vi "subVI_CurrentSourcing.vi"(4 "error in":errorcluster caption="에러 입력", 5 "stop (T)":bool=TRUE caption="정지(T)", 6 "timeout (s)":dbl=10.0 caption="타임아웃(초)" format="%0.2f", 7 "Curr set val":dbl[](array[numeric]) caption="배열" format="%0.2f") -> (0 "error out":errorcluster caption="에러 출력", 3 "task out":refnum<k21> caption="태스크 출력")   [LabVIEW 2016]
doc: "NI-DAQmx를 사용하여 태스크를 생성, 편집, 실행합니다. NI-DAQmx가 지원하는 디바이스의 완전한 리스트는 NI-DAQ Readme를 참조하십시오.\n\n이 익스프레스 VI를 블록다이어그램에 놓으면 DAQ 어시스턴트가 시작되어 새로운 태스크를 생성합니다, 태스크를 생성한 후, DAQ 어시스턴트 익스프레스 VI를 더블 클릭하여 해당 태스크를 편집할 수 있습니다. 연속적인 측정 또는 생성을 위해서는 DAQ 어시스턴트 익스프레스 주위에 while 루프를 놓습니다.\n\n연속적인 단일 포인트 입력 또는 출력의 경우 DAQ 어시스턴트 익스프레스 VI는 최적의 성능을 제공하지 않을 수도 있습니다. 높은 성능을 가진 단일 포인트 I/O 어플리케이션을 생성하는 기술에 대한 예제는 examples\\DAQmx\\Analog In\\Measure Voltage.llb의 Cont Acq&Graph Voltage-Single Point Optimization VI를 참조하십시오."
uses:
  <vilib>/DAQmx/write.llb/DAQmx Write.vi
  <vilib>/DAQmx/write.llb/DAQmx Write (Analog 1D DBL NChan 1Samp).vi
  <vilib>/DAQmx/create/channels.llb/DAQmx Create Channel (AO-Current-Basic).vi
  <vilib>/DAQmx/miscellaneous.llb/DAQmx Fill In Error Info.vi
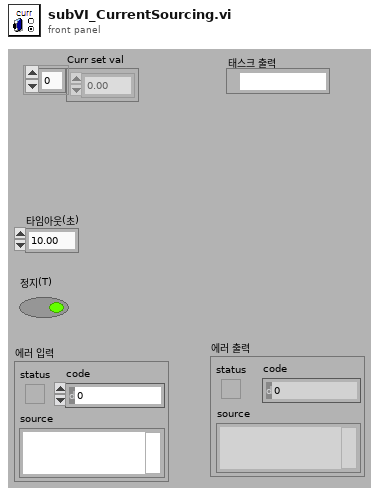
[diagram p1: front panel]
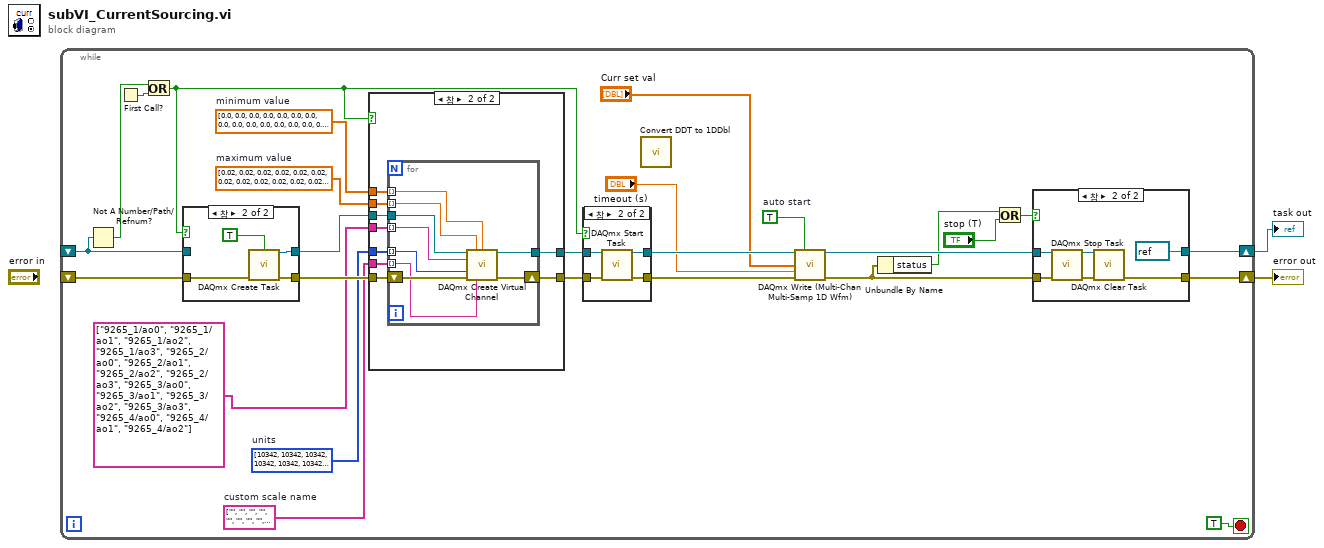
[diagram p0: block diagram]
diagram:
  n1 = while {
    shift-right: [w11] -> w1
    shift-left: _ -> [w26]
    shift-right: [w9] -> w2
    shift-left: _ -> [w27]
    stop <- TRUE stop-if-true
    w13 = TRUE  # auto start
    w19 = string[] ["", "", "", "", "", "", "", "", "", "", "", "", "", "", "", ""]  # custom scale name
    w20 = i32[] [10342, 10342, 10342, 10342, 10342, 10342, 10342, 10342, 10342, 10342, 10342, 10342, 10342, 10342, 10342, 10342] items=["Amps"=10342, "From Custom Scale"=10065]  # units
    w21 = dbl[] [0.02, 0.02, 0.02, 0.02, 0.02, 0.02, 0.02, 0.02, 0.02, 0.02, 0.02, 0.02, 0.02, 0.02, 0.02, 0.02]  # maximum value
    w22 = dbl[] [0.0, 0.0, 0.0, 0.0, 0.0, 0.0, 0.0, 0.0, 0.0, 0.0, 0.0, 0.0, 0.0, 0.0, 0.0, 0.0]  # minimum value
    n2 = Not A Number/Path/Refnum?(number/path/refnum=w26) -> (NaN/Path/Refnum?=w25:bool)
    n3 = First Call?() -> (First Call?: T/F=w28:bool)
    n4 = Or(x=w25, y=w28) -> (x .or. y?=w18:bool)
    n5 = case "케이스 구조" shown="참" w18 {
      tunnel: [w65 w69] -> w24
      tunnel: w26 -> [w65 _]
      tunnel: [w64 w68] -> w23
      tunnel: w27 -> [w64 w66]
      frame False {
      }
      frame True {
        n6 = call <vilib>:"DAQmx Create Task.vi"("auto cleanup"=TRUE, "error in"=w66) -> ("task out"=w69:refnum<k21>, "error out"=w68:errorcluster)  [unwired: 12 in]
      }
    }
    n7 = case "케이스 구조" shown="참" w18 {
      tunnel: [w45 w52] -> w17
      tunnel: w24 -> [w45 w54]
      tunnel: [w44 w51] -> w16
      tunnel: w23 -> [w44 w53]
      tunnel: w22 -> [_ w50]
      tunnel: w21 -> [_ w49]
      tunnel: tag[] ["9265_1/ao0", "9265_1/ao1", "9265_1/ao2", "9265_1/ao3", "9265_2/ao0", "9265_2/ao1", "9265_2/ao2", "9265_2/ao3", "9265_3/ao0", "9265_3/ao1", "9265_3/ao2", "9265_3/ao3", "9265_4/ao0", "9265_4/ao1", "9265_4/ao2"] -> [_ w48]
      tunnel: w20 -> [_ w47]
      tunnel: w19 -> [_ w46]
      frame False {
      }
      frame True {
        n8 = for "For 루프" {
          tunnel: w54 -> [w63]
          tunnel: [w61] -> w52
          tunnel: w50 -> [w59] mode=indexing
          tunnel: w49 -> [w58] mode=indexing
          tunnel: w48 -> [w57] mode=indexing
          tunnel: w47 -> [w56] mode=indexing
          tunnel: w46 -> [w55] mode=indexing
          shift-right: [w60] -> w51
          shift-left: w53 -> [w62]
          n9 = call-poly <vilib>:"DAQmx Create Virtual Channel.vi"("task in"=w63, "maximum value"=w58, "minimum value"=w59, "physical channels"=w57, "units"=w56, "error in"=w62, "custom scale name"=w55) -> ("task out"=w61:refnum<k21>, "error out"=w60:errorcluster)  [unwired: 7 in]
        }
      }
    }
    n10 = case "케이스 구조" shown="참" w18 {
      tunnel: [w39 w42] -> w15
      tunnel: w17 -> [w39 w43]
      tunnel: [w38 w40] -> w14
      tunnel: w16 -> [w38 w41]
      frame False {
      }
      frame True {
        n11 = call <vilib>:"DAQmx Start Task.vi"("task/channels in"=w43, "error in"=w41) -> ("task out"=w42:refnum<k21>, "error out"=w40:errorcluster)  [unwired: 12 in]
      }
    }
    n12 = call <vilib>:"Convert DDT to 1DDbl.vi"() -> ()  [unwired: 4 in, 1 out]
    n13 = call-poly "DAQmx Write (Multi-Chan Multi-Samp 1D Wfm).vi"("task/channels in"=w15, "auto start"=w13, "data"="Curr set val", "timeout"="timeout (s)", "error in"=w14) -> ("task out"=w10:refnum<k21>, "error out"=w8:errorcluster)  [unwired: 8 in, 1 out]
    n14 = Unbundle By Name(w8) -> ("status"=w7:bool)
    n15 = Or(x=w7, y="stop (T)") -> (x .or. y?=w5:bool)
    n16 = case "케이스 구조" shown="참" w5 {
      tunnel: [w31 refnum<k21> refnum ("task in")] -> w11
      tunnel: w10 -> [w31 w37]
      tunnel: [w30 w34] -> w9
      tunnel: w8 -> [w30 w36]
      frame False {
      }
      frame True {
        n17 = call <vilib>:"DAQmx Stop Task.vi"("task/channels in"=w37, "error in"=w36) -> ("task out"=w33:refnum<k21>, "error out"=w35:errorcluster)  [unwired: 12 in]
        n18 = call <vilib>:"DAQmx Clear Task.vi"("task in"=w33, "error in"=w35) -> ("error out"=w34:errorcluster)  [unwired: 13 in]
      }
    }
  }
  "error out" <- w2
  "task out" <- w1
